vi "Untitled 1.vi"() -> ()   [LabVIEW 2020]
uses:
  http-client.lvclass
  Response Headers/Response Headers.lvclass
panel:
  out "status code":u16
  out "header":refnum<class "Response Headers.lvclass">
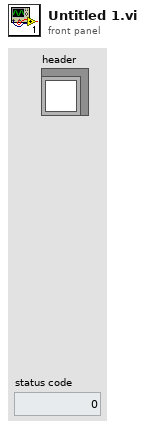
[diagram p1: front panel]
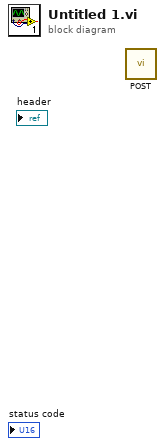
[diagram p0: block diagram]
diagram:
  n1 = call "POST.vi"() -> ()  [unwired: 7 in, 5 out]
